vi "execute.vi"(8 "error in (no error)":errorcluster, 11 "BuyStock in":refnum<class "BuyStock.lvclass">) -> (0 "error out":errorcluster, 3 "BuyStock out":refnum<class "BuyStock.lvclass">)   [LabVIEW 2017, in "BuyStock.lvclass"]
uses:
  BuyStock.lvclass
  BuyStock.lvclass/BuyStock.ctl
  Stock Class/Stock.lvclass
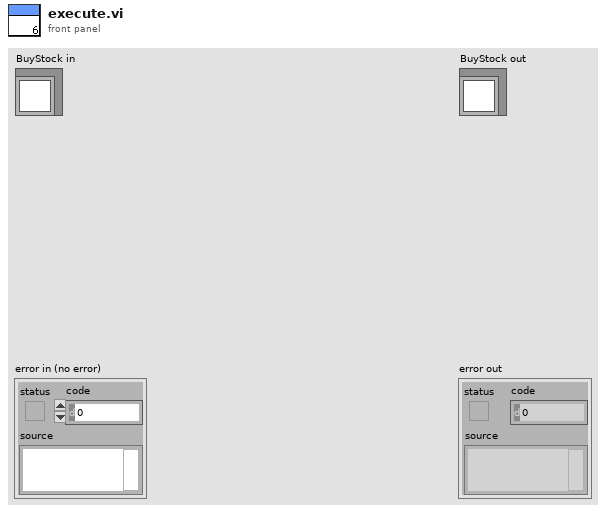
[diagram p1: front panel]
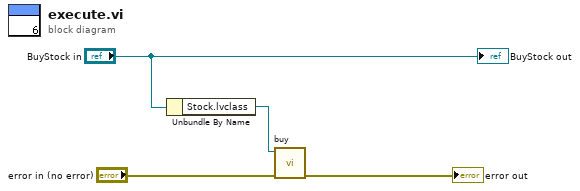
[diagram p0: block diagram]
diagram:
  n1 = Unbundle By Name("BuyStock in") -> ("Stock.lvclass"=w1:refnum<class "Stock.lvclass">)
  n2 = call "buy.vi"("error in (no error)"="error in (no error)", "Stock in"=w1) -> ("error out"=→"error out":errorcluster)  [unwired: 8 in, 1 out]
  "BuyStock out" <- "BuyStock in"
